vi "joystick-encoding-booleans.vi"() -> ()   [LabVIEW 2018]
panel:
  out "String":string
  out "number":u32
  in  "Button Array":bool[](array[boolean])
  # "1\n\n2\n\n3\n\n4\n\n5\n\n6\n\n7\n\n8\n\n9\n\n10\n\n11\n\n12"
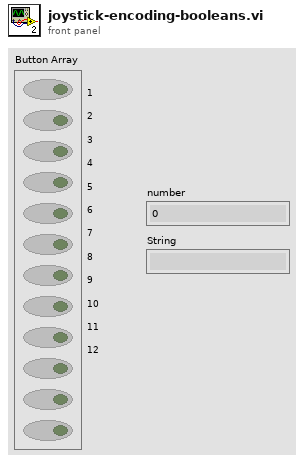
[diagram p1: front panel]
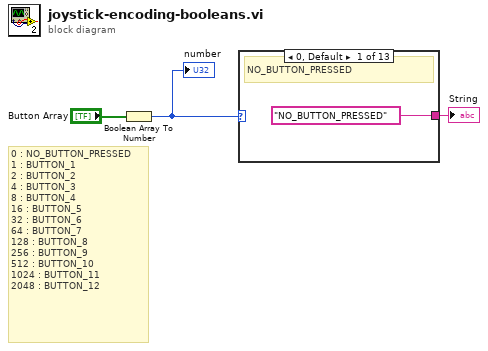
[diagram p0: block diagram]
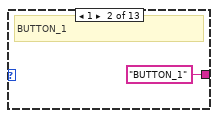
[diagram p2: hidden frame]
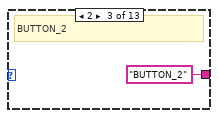
[diagram p3: hidden frame]
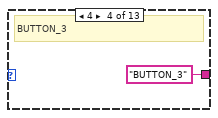
[diagram p4: hidden frame]
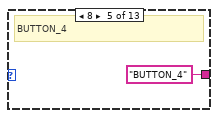
[diagram p5: hidden frame]
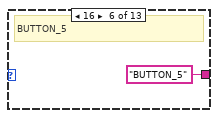
[diagram p6: hidden frame]
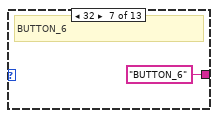
[diagram p7: hidden frame]
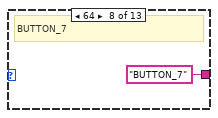
[diagram p8: hidden frame]
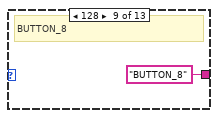
[diagram p9: hidden frame]
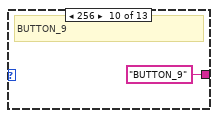
[diagram p10: hidden frame]
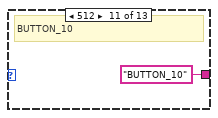
[diagram p11: hidden frame]
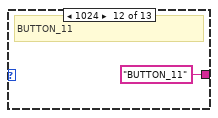
[diagram p12: hidden frame]
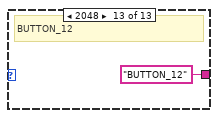
[diagram p13: hidden frame]
diagram:
  # "0 : NO_BUTTON_PRESSED\n1 : BUTTON_1\n2 : BUTTON_2\n4 : BUTTON_3\n8 : BUTTON_4\n16 : BUTTON_5\n32 : BUTTON_6\n64 : BUTTON_7\n128 : BUTTON_8\n256 : BUTTON_9\n512 : BUTTON_10\n1024 : BUTTON_11\n2048 : BUTTON_12"
  n1 = Boolean Array To Number(Boolean array="Button Array") -> (number=w2:u32)
  "number" <- w2
  n2 = case shown="0, Default" w2 {
    tunnel: ["NO_BUTTON_PRESSED" "BUTTON_1" "BUTTON_2" "BUTTON_3" "BUTTON_4" "BUTTON_5" "BUTTON_6" "BUTTON_7" "BUTTON_8" "BUTTON_9" "BUTTON_10" "BUTTON_11" "BUTTON_12"] -> w1
    frame 0, Default {
      # "NO_BUTTON_PRESSED"
    }
    frame 1 {
      # "BUTTON_1"
    }
    frame 2 {
      # "BUTTON_2"
    }
    frame 4 {
      # "BUTTON_3"
    }
    frame 8 {
      # "BUTTON_4"
    }
    frame 16 {
      # "BUTTON_5"
    }
    frame 32 {
      # "BUTTON_6"
    }
    frame 64 {
      # "BUTTON_7"
    }
    frame 128 {
      # "BUTTON_8"
    }
    frame 256 {
      # "BUTTON_9"
    }
    frame 512 {
      # "BUTTON_10"
    }
    frame 1024 {
      # "BUTTON_11"
    }
    frame 2048 {
      # "BUTTON_12"
    }
  }
  "String" <- w1
